vi "Read Measurements.vi"(8 "error in (no error)":errorcluster, 11 "ACIR Instrument in":refnum<class "ACIR Instrument.lvclass">) -> (0 "error out":errorcluster, 2 "Measurements":T1[](array[typedef]) {"Lower limit" format="%#_4p"; "Upper limit" format="%#_4p"}, 3 "ACIR Instrument out":refnum<class "ACIR Instrument.lvclass">)   [LabVIEW 2025, in "ACIR.lvlib" / "ACIR Instrument.lvclass"]
uses:
  ACIR Instrument.lvclass
  C:/Users/Public/Documents/Sandia National Labs/TSS Plugin/Abstract Engine.lvlibp/Plugin/Abstract/Abstract Instrument/Abstract Instrument.lvclass
  Users/Public/Documents/Sandia National Labs/TSS Plugin/Abstract Engine.lvlibp/Plugin/Abstract/Abstract Instrument/Channel.ctl
  Users/Public/Documents/Sandia National Labs/TSS Plugin/Abstract Engine.lvlibp/Plugin/Abstract/Abstract Instrument/Abstract Instrument.lvclass
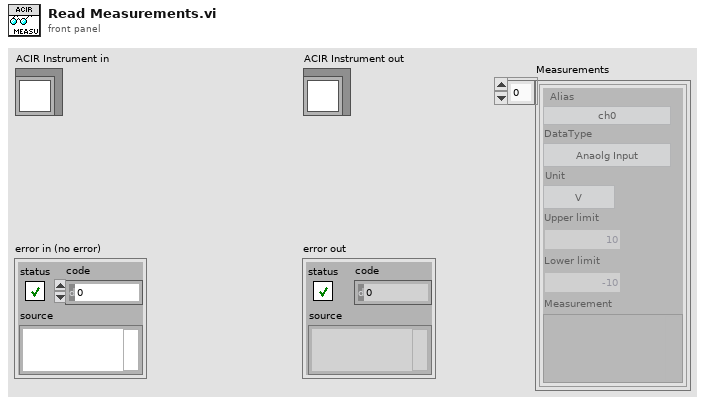
[diagram p1: front panel]
types:
  T1 = typedef "Abstract Engine.lvlibp/Abstract Instrument.lvclass/Channel.ctl" = cluster{"Alias":string, "DataType":enum16{"Anaolg Input", "Waveform"}, "Unit":enum16{"---", "V", "A", "Ohm", "Hz", "uF", "degC", "deg"}, "Upper limit":dbl, "Lower limit":dbl, "Measurement":variant}
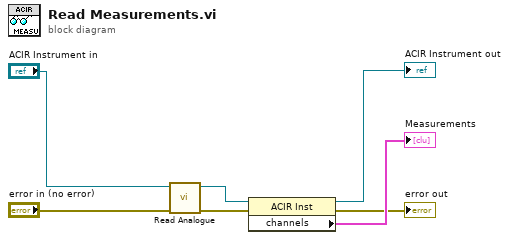
[diagram p0: block diagram]
diagram:
  n1 = call-dynamic "Read Analogue.vi"("error in (no error)"="error in (no error)", "ACIR Instrument"="ACIR Instrument in") -> ("error out"=w3:errorcluster, "ACIR Instrument out"=w5:refnum<class "ACIR Instrument.lvclass">)  [unwired: 7 in, 1 out]
  n2 = property class="ACIR Inst"(reference=w5, error in=w3) -> (reference out=→"ACIR Instrument out":refnum<class "ACIR Instrument.lvclass">, error out=→"error out":errorcluster, "channels"=→"Measurements":T1[])
